vi "IDS_system_isTestChannelEnabled.vi"(8 "error in (no error)":errorcluster, 11 "deviceHandle":i32) -> (0 "error out":errorcluster, 2 "enabled out":bool, 3 "deviceHandle out":i32)   [LabVIEW 2016]
doc: "int IDS_DLL IDS_laser_isEnabled(bool * enabled);"
panel:
  in  "enabled":bool
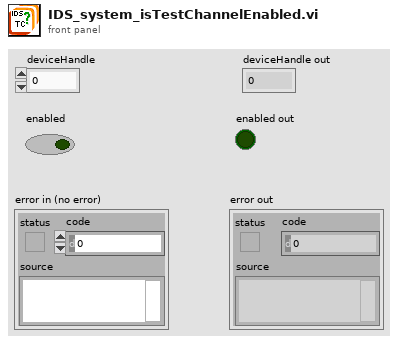
[diagram p1: front panel]
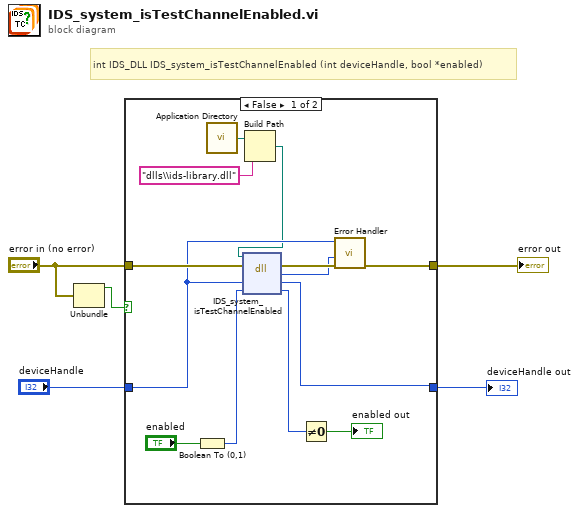
[diagram p0: block diagram]
diagram:
  # "int IDS_DLL IDS_system_isTestChannelEnabled (int deviceHandle, bool *enabled)"
  n1 = Unbundle("error in (no error)") -> ("status"=w1:bool)  [unwired: 2 out]
  n2 = case shown="False" w1 {
    tunnel: "error in (no error)" -> [w15 w20]
    tunnel: [w16 w20] -> w5
    tunnel: "deviceHandle" -> [w10 w19]
    tunnel: [w11 w19] -> w3
    frame False {
      n3 = Boolean To (0,1)(Boolean="enabled") -> (0, 1=w13:i16)
      n4 = call <vilib>:"Application Directory.vi"() -> ("Application Directory"=w8:path)
      n5 = Build Path(base path=w8, name or relative path="dlls\\ids-library.dll" ("ipAddress")) -> (appended path=w6:path)
      n6 = dll-call lib="C:/Users/matheus/Desktop/LabVIEW_Draft_V1.6.0/dlls/ids-library.*" fn="IDS_system_isTestChannelEnabled"(path in=w6, error in=w15, "deviceHandle"=w10, "enabled"=w13) -> (error out=w14:errorcluster, "return type"=w9:i32, "deviceHandle"=w11:i32, "enabled"=w12:u8)  [unwired: 1 in, 1 out]
      n7 = Not Equal To 0?(x=w12) -> (x != 0?=→"enabled out":bool)
      n8 = call "Error Handler.vi"("error in (no error)"=w14, "error code"=w9, "deviceHandle"=w10) -> ("error out"=w16:errorcluster)  [unwired: 7 in, 1 out]
    }
    frame True {
    }
  }
  "error out" <- w5
  "deviceHandle out" <- w3
